vi "COPY.vi"(6 "CSV?":bool, 7 "column name(s) (empty=ALL)":string, 8 "error in (no error)":errorcluster, 9 "buffer":string, 10 "table name":string, 11 "PQ Connection in":refnum<class "PQ Connection.lvclass">) -> (0 "error out":errorcluster, 3 "PQ Connection out":refnum<class "PQ Connection.lvclass">)   [LabVIEW 2016, in "PQ Connection.lvclass"]
uses:
  PQ Connection.lvclass
  PQ Connection.lvclass/PQ Connection.ctl
  Result/PQ Result.lvclass/PQ Result.ctl
  Result/PQ Result.lvclass
  libpq.dll
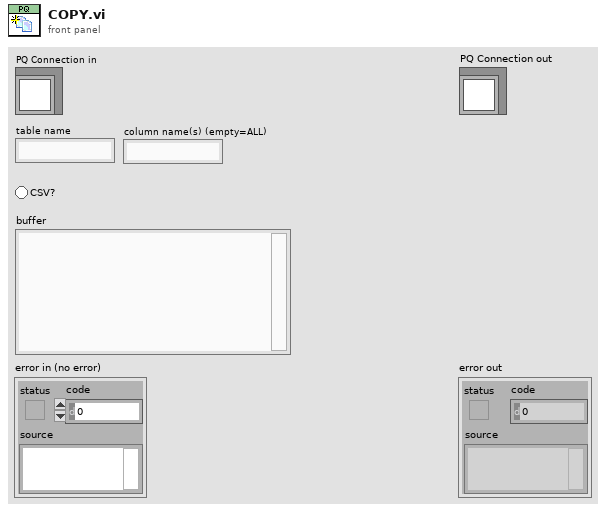
[diagram p1: front panel]
types:
  T1 = typedef "PQ Result.lvclass/Result Status.ctl" = enum32{"PGRES_EMPTY_QUERY", "PGRES_COMMAND_OK", "PGRES_TUPLES_OK", "PGRES_COPY_OUT", "PGRES_COPY_IN", "PGRES_BAD_RESPONSE", "PGRES_NONFATAL_ERROR", "PGRES_FATAL_ERROR", "PGRES_COPY_BOTH", "PGRES_SINGLE_TUPLE"}
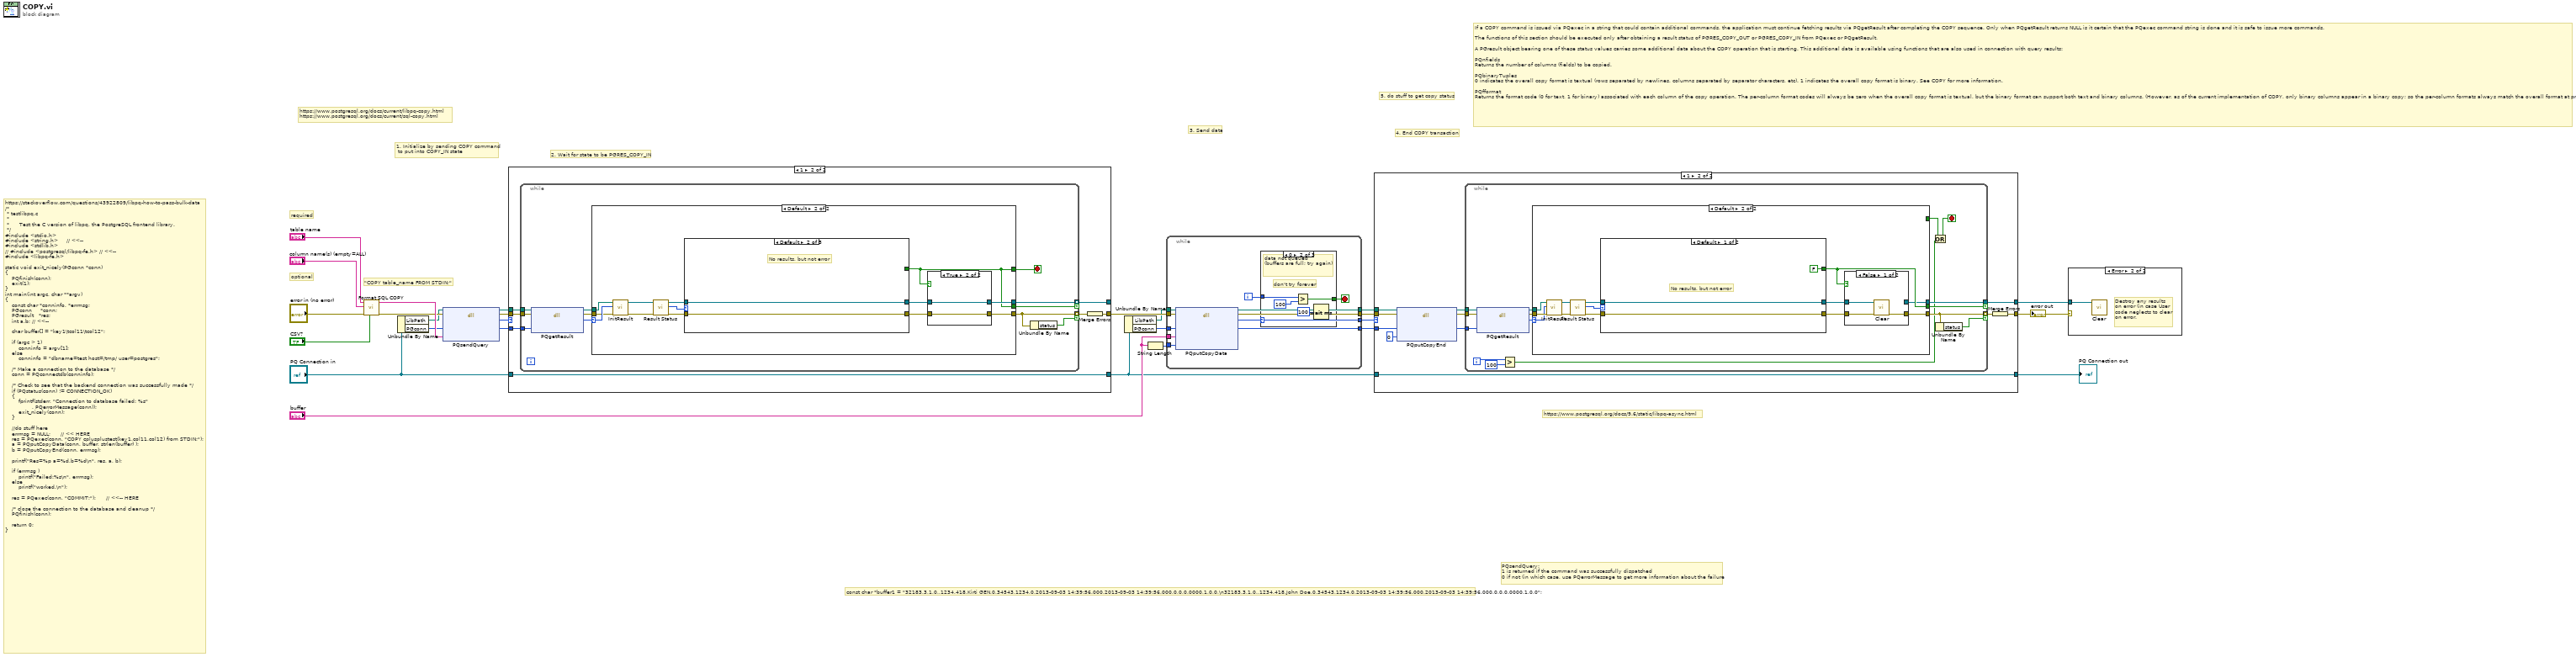
[diagram p0: block diagram]
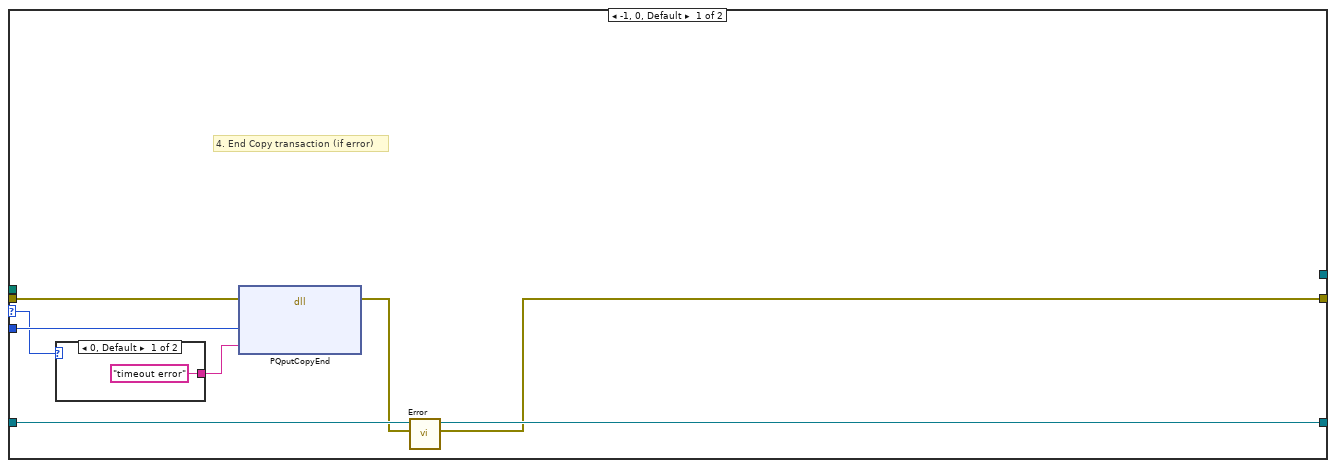
[diagram p2: hidden frame]
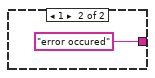
[diagram p3: hidden frame]
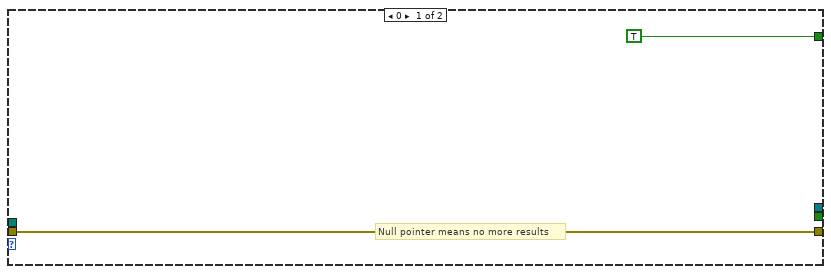
[diagram p4: hidden frame]
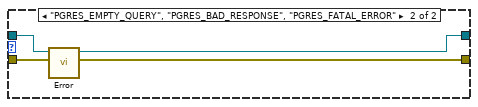
[diagram p5: hidden frame]
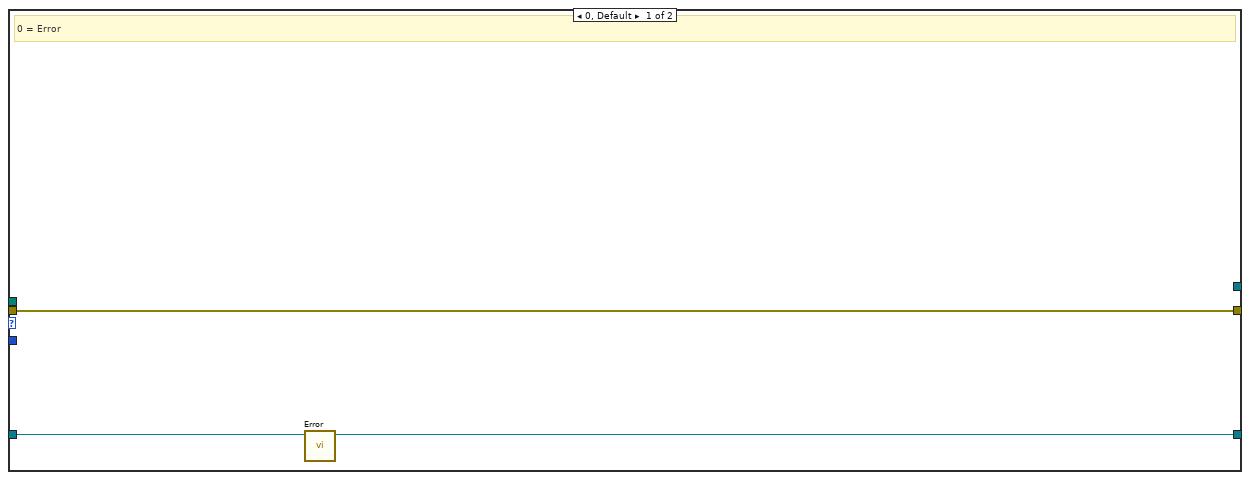
[diagram p7: hidden frame]
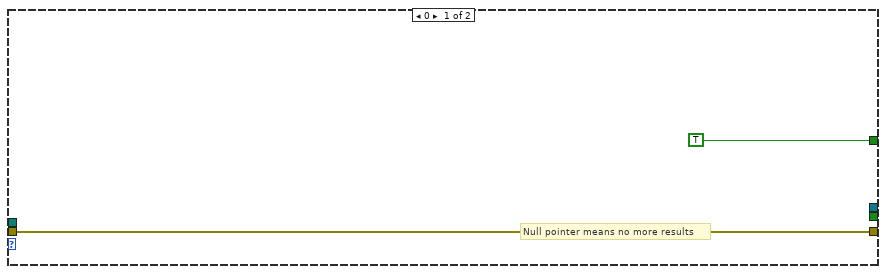
[diagram p8: hidden frame]
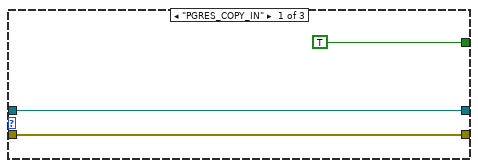
[diagram p9: hidden frame]
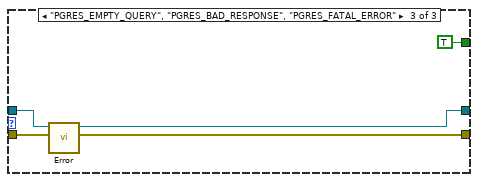
[diagram p10: hidden frame]
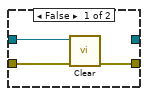
[diagram p11: hidden frame]
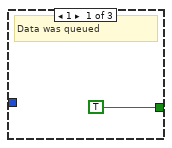
[diagram p12: hidden frame]
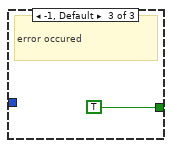
[diagram p13: hidden frame]
diagram:
  # "\"COPY table_name FROM STDIN;\""
  # "4. End COPY transaction"
  # "https://www.postgresql.org/docs/9.6/static/libpq-async.html"
  # "If a COPY command is issued via PQexec in a string that could contain additional commands, the application must continue fetching results via PQgetResult after completing the COPY sequence. Only when PQgetResult returns NULL is it certain that the PQexec command string is done and it is safe to issue more commands.\n\nThe functions of this section should be executed only after obtaining a result status of PGRES_COPY_OUT or PGRES_COPY_IN from PQexec or PQgetResult.\n\nA PGresult object bearing one of these status values carries some additional data about the COPY operation that is starting. This additional data is available using functions that are also used in connection with query results:\n\nPQnfields\nReturns the number of columns (fields) to be copied.\n\nPQbinaryTuples\n0 indicates the overall copy format is textual (rows separated by newlines, columns separated by separator characters, etc). 1 indicates the overall copy format is binary. See COPY for more information.\n\nPQfformat\nReturns the format code (0 for text, 1 for binary) associated with each column of the copy operation. The per-column format codes will always be zero when the overall copy format is textual, but the binary format can support both text and binary columns. (However, as of the current implementation of COPY, only binary columns appear in a binary copy; so the per-column formats always match the overall format at present.)"
  # "5. do stuff to get copy status"
  # "3. Send data"
  # "2. Wait for state to be PGRES_COPY_IN"
  # "1. Initialize by sending COPY command\n to put into COPY_IN state"
  # "optional"
  # "required"
  # "https://www.postgresql.org/docs/current/libpq-copy.html\nhttps://www.postgresql.org/docs/current/sql-copy.html"
  # "PQsendQuery:\n1 is returned if the command was successfully dispatched\n0 if not (in which case, use PQerrorMessage to get more information about the failure"
  # "const char *buffer1 = \"32183,3,1,0,,1234,418,Kirti GEN,0,34543,1234,0,2013-09-03 14:39:56.000,2013-09-03 14:39:56.000,0,0,0.0000,1,0,0,\\n32183,3,1,0,,1234,418,John Doe,0,34543,1234,0,2013-09-03 14:39:56.000,2013-09-03 14:39:56.000,0,0,0.0000,1,0,0\";"
  # "https://stackoverflow.com/questions/43922809/libpq-how-to-pass-bulk-data\n/*\n * testlibpq.c\n *\n *      Test the C version of libpq, the PostgreSQL frontend library.\n */\n#include <stdio.h>\n#include <string.h>     // <<--\n#include <stdlib.h>\n// #include <postgresql/libpq-fe.h> // <<--\n#include <libpq-fe.h>\n\nstatic void exit_nicely(PGconn *conn)\n{\n    PQfinish(conn);\n    exit(1);\n}\nint main(int argc, char **argv)\n{\n    const char *conninfo, *errmsg;\n    PGconn     *conn;\n    PGresult   *res;\n    int a,b; // <<--\n\n    char buffer[] = \"key1\\tcol11\\tcol12\";\n\n    if (argc > 1)\n        conninfo = argv[1];\n    else\n        conninfo = \"dbname=test host=/tmp/ user=postgres\";\n\n    /* Make a connection to the database */\n    conn = PQconnectdb(conninfo);\n\n    /* Check to see that the backend connection was successfully made */\n    if (PQstatus(conn) != CONNECTION_OK)\n    {\n        fprintf(stderr, \"Connection to database failed: %s\"\n                , PQerrorMessage(conn));\n        exit_nicely(conn);\n    }\n\n    //do stuff here\n    errmsg = NULL;      // << HERE\n    res = PQexec(conn, \"COPY cplusplustest(key1,col11,col12) from STDIN;\");\n    a = PQputCopyData(conn, buffer, strlen(buffer) );\n    b = PQputCopyEnd(conn, errmsg);\n\n    printf(\"Res=%p a=%d,b=%d\\n\", res, a, b);\n\n    if (errmsg )\n        printf(\"Failed:%s\\n\", errmsg);\n    else\n        printf(\"worked.\\n\");\n\n    res = PQexec(conn, \"COMMIT;\");      // <<-- HERE\n\n    /* close the connection to the database and cleanup */\n    PQfinish(conn);\n\n    return 0;\n}"
  n1 = call "Format SQL COPY.vi"("CSV?"="CSV?", "error in (no error)"="error in (no error)", "column name(s)"="column name(s) (empty=ALL)", "table name"="table name") -> ("error out"=w10:errorcluster, "COPY SQL"=w20:string)  [unwired: 6 in]
  n2 = Unbundle By Name("PQ Connection in") -> ("LibPath"=w5:path, "PGconn"=w19:u32)
  n3 = dll-call lib="C:/Users/patrick/Documents/GitHub/pq-labview-levylab/Connection/libpq.dll" fn="PQsendQuery" ("libpq.*:PQexec")(path in=w5, error in=w10, "PGconn"=w19, "command"=w20) -> (path out=w4:path, error out=w18:errorcluster, "OK?"=w17:u32, "PGconn"=w16:u32)  [unwired: 2 in]
  n4 = case shown="1" w17 {
    tunnel: w18 -> [w27 w36]
    tunnel: [_ w35] -> _
    tunnel: [w27 w31] -> w14
    tunnel: "PQ Connection in" -> [w29 w32]
    tunnel: [w28 w32] -> w15
    tunnel: w16 -> [_ w33]
    tunnel: w4 -> [_ w30]
    frame 0, Default {
      # "0 = Error"
      n5 = call "Error.vi"("PQ Connection in"=w29) -> ("PQ Connection out"=w28:refnum<class "PQ Connection.lvclass">)  [unwired: 9 in, 1 out]
    }
    frame 1 {
      n6 = while {
        tunnel: [w45] -> w35 mode=indexing if=w46
        tunnel: w33 -> [w47]
        tunnel: w36 -> [w42]
        tunnel: [w40] -> w34 mode=indexing if=w39
        tunnel: w30 -> [w38]
        stop <- w43 stop-if-true
        n7 = dll-call lib="C:/Users/patrick/Documents/GitHub/pq-labview-levylab/Connection/libpq.dll" fn="PQgetResult" ("libpq.*:PQexec")(path in=w38, error in=w42, "PGconn"=w47) -> (path out=w37:path, error out=w41:errorcluster, "PQresult"=w44:u32)  [unwired: 2 in]
        n8 = case shown="Default" w44 {
          selector: w44 -> [_ w53]
          tunnel: w41 -> [w49 w51]
          tunnel: [_ w56] -> w46
          tunnel: [_ w61] -> w45
          tunnel: [w49 w59] -> w40
          tunnel: [TRUE w56] -> w43
          tunnel: w37 -> [_ w54]
          frame 0 {
            # "Null pointer means no more results"
          }
          frame Default {
            n9 = call "InitResult.vi"("error in (no error)"=w51, "PGresult"=w53, "LibPath"=w54) -> ("error out"=w50:errorcluster, "PQ Result out"=w52:refnum<class "PQ Result.lvclass">)  [unwired: 7 in]
            n10 = call "Result Status.vi"("error in (no error)"=w50, "PQ Result in"=w52) -> ("error out"=w57:errorcluster, "Result Status"=w55:T1, "PQ Result out"=w58:refnum<class "PQ Result.lvclass">)  [unwired: 7 in]
            n11 = case shown="Default" w55 {
              tunnel: [w64 w66 w69] -> w62
              tunnel: w58 -> [w64 w66 w72]
              tunnel: w57 -> [w65 w67 w71]
              tunnel: [w65 w67 w70] -> w60
              tunnel: [TRUE _ TRUE] -> w56
              frame "PGRES_COPY_IN" {
              }
              frame Default {
                # "No results, but not error"
              }
              frame "PGRES_EMPTY_QUERY", "PGRES_BAD_RESPONSE", "PGRES_FATAL_ERROR" {
                n12 = call "Error.vi"("error in (no error)"=w71, "PQ Result  In"=w72) -> ("error out"=w70:errorcluster, "PQ Result"=w69:refnum<class "PQ Result.lvclass">)  [unwired: 8 in]
              }
            }
            n13 = case shown="True" w56 {
              tunnel: w62 -> [w75 w77]
              tunnel: [_ w77] -> w61
              tunnel: w60 -> [w74 w76]
              tunnel: [w73 w76] -> w59
              frame False {
                n14 = call "Clear.vi"("error in (no error)"=w74, "PQ Result  in"=w75) -> ("error out"=w73:errorcluster)  [unwired: 9 in]
              }
              frame True {
              }
            }
          }
        }
        n15 = Unbundle By Name(w40) -> ("status"=w39:bool)
      }
      n16 = Merge Errors(w34) -> (w31:errorcluster)
    }
  }
  n17 = Unbundle By Name(w15) -> ("LibPath"=w2:path, "PGconn"=w21:u32)
  n18 = String Length(string="buffer") -> (length=w24:i32)
  n19 = while {
    tunnel: "buffer" -> [w84]
    tunnel: w21 -> [w88]
    tunnel: [w87] -> w25
    tunnel: w24 -> [w83]
    tunnel: [w82] -> w23
    tunnel: w14 -> [w86]
    tunnel: [w85] -> w13
    tunnel: [w79] -> w3
    tunnel: w2 -> [w78]
    i -> [w80]
    stop <- w81 stop-if-true
    n20 = dll-call lib="C:/Users/patrick/Documents/GitHub/pq-labview-levylab/Connection/libpq.dll" fn="PQputCopyData" ("libpq.*:PQexec")(path in=w78, error in=w86, "PGconn"=w88, "buffer"=w84, "nbytes"=w83) -> (path out=w79:path, error out=w85:errorcluster, "OK?"=w82:i32, "PGconn"=w87:u32)  [unwired: 3 in]
    n21 = case shown="0" w82 {
      tunnel: [TRUE w91 TRUE] -> w81
      tunnel: w80 -> [_ w93 _]
      frame 1 {
        # "Data was queued"
      }
      frame 0 {
        # "don't try forever"
        # "data not queued\n(buffers are full; try again)"
        n22 = Greater?(x=w93, y=100) -> (0:w91:bool)
        n23 = Wait (ms)(milliseconds to wait=u32 100) -> ()  [unwired: 1 out]
      }
      frame -1, Default {
        # "error occured"
      }
    }
  }
  n24 = case shown="1" w23 {
    selector: w23 -> [w96 _]
    tunnel: w13 -> [w99 w111]
    tunnel: [_ w115] -> w26
    tunnel: [w100 w112] -> w12
    tunnel: w15 -> [w102 w113]
    tunnel: [w101 w113] -> w6
    tunnel: w25 -> [w98 w108]
    tunnel: w3 -> [_ w105]
    frame -1, 0, Default {
      # "4. End Copy transaction (if error)"
      n25 = case shown="0, Default" w96 {
        tunnel: ["timeout error" "error occured"] -> w95
        frame 0, Default {
        }
        frame 1 {
        }
      }
      n26 = dll-call lib="C:/Users/patrick/Documents/GitHub/pq-labview-levylab/Connection/libpq.dll" fn="PQputCopyEnd" ("libpq.*:PQexec")(error in=w99, "PGconn"=w98, "errormsg"=w95) -> (error out=w97:errorcluster)  [unwired: 5 in, 1 out]
      n27 = call "Error.vi"("error in (no error)"=w97, "PQ Connection in"=w102) -> ("error out"=w100:errorcluster, "PQ Connection out"=w101:refnum<class "PQ Connection.lvclass">)  [unwired: 8 in]
    }
    frame 1 {
      n28 = dll-call lib="C:/Users/patrick/Documents/GitHub/pq-labview-levylab/Connection/libpq.dll" fn="PQputCopyEnd" ("libpq.*:PQexec")(path in=w105, error in=w111, "PGconn"=w108, "errormsg"=u32 0) -> (path out=w106:path, error out=w110:errorcluster, "PGconn"=w109:u32)  [unwired: 3 in]
      n29 = while {
        tunnel: [w128] -> w115 if=w129
        tunnel: w109 -> [w130]
        tunnel: w110 -> [w126]
        tunnel: [w123] -> w114 mode=indexing if=w124
        tunnel: w106 -> [w117]
        i -> [w122]
        stop <- w118 stop-if-true
        n30 = dll-call lib="C:/Users/patrick/Documents/GitHub/pq-labview-levylab/Connection/libpq.dll" fn="PQgetResult" ("libpq.*:PQexec")(path in=w117, error in=w126, "PGconn"=w130) -> (path out=w116:path, error out=w125:errorcluster, "PQresult"=w127:u32)  [unwired: 2 in]
        n31 = Greater?(x=w122, y=100) -> (0:w120:bool)
        n32 = case shown="Default" w127 {
          selector: w127 -> [_ w135]
          tunnel: w125 -> [w132 w137]
          tunnel: [_ w145] -> w129
          tunnel: [_ w143] -> w128
          tunnel: [w132 w141] -> w123
          tunnel: [TRUE _] -> w119
          tunnel: w116 -> [_ w134]
          frame 0 {
            # "Null pointer means no more results"
          }
          frame Default {
            n33 = call "InitResult.vi"("error in (no error)"=w137, "PGresult"=w135, "LibPath"=w134) -> ("error out"=w136:errorcluster, "PQ Result out"=w133:refnum<class "PQ Result.lvclass">)  [unwired: 7 in]
            n34 = call "Result Status.vi"("error in (no error)"=w136, "PQ Result in"=w133) -> ("error out"=w139:errorcluster, "Result Status"=w138:T1, "PQ Result out"=w140:refnum<class "PQ Result.lvclass">)  [unwired: 7 in]
            n35 = case shown="Default" w138 {
              tunnel: [w147 w149] -> w144
              tunnel: w140 -> [w147 w152]
              tunnel: w139 -> [w148 w151]
              tunnel: [w148 w150] -> w142
              tunnel: [FALSE _] -> w145
              frame Default {
                # "No results, but not error"
              }
              frame "PGRES_EMPTY_QUERY", "PGRES_BAD_RESPONSE", "PGRES_FATAL_ERROR" {
                n36 = call "Error.vi"("error in (no error)"=w151, "PQ Result  In"=w152) -> ("error out"=w150:errorcluster, "PQ Result"=w149:refnum<class "PQ Result.lvclass">)  [unwired: 8 in]
              }
            }
            n37 = case shown="False" w145 {
              tunnel: w144 -> [w155 w157]
              tunnel: [_ w157] -> w143
              tunnel: w142 -> [w154 w156]
              tunnel: [w153 w156] -> w141
              frame False {
                n38 = call "Clear.vi"("error in (no error)"=w154, "PQ Result  in"=w155) -> ("error out"=w153:errorcluster)  [unwired: 9 in]
              }
              frame True {
              }
            }
          }
        }
        n39 = Or(x=w119, y=w120) -> (x .or. y?=w118:bool)
        n40 = Unbundle By Name(w123) -> ("status"=w124:bool)
      }
      n41 = Merge Errors(w114) -> (w112:errorcluster)
    }
  }
  "error out" <- w12
  "PQ Connection out" <- w6
  n42 = case shown="Error" w12 {
    tunnel: w26 -> [_ w158]
    frame No Error {
    }
    frame Error {
      # "Destroy any results\non error (in case User\ncode neglects to clear\non error."
      n43 = call "Clear.vi"("PQ Result  in"=w158) -> ()  [unwired: 10 in, 1 out]
    }
  }
